vi "Hausmodell.Rücklauftemperatur.vi"(8 "Error IN":errorcluster, 10 "Vorlauftemperatur Heizkreislauf [°C]":dbl, 11 "Hausmodell IN":refnum<data-value>) -> (0 "Error OUT":errorcluster, 3 "Hausmodell OUT":refnum<data-value>)   [LabVIEW 2016, in "Hausmodell.lvclass"]
uses:
  Hausmodell.lvclass
  Hausmodell.lvclass/Hausmodell.ctl
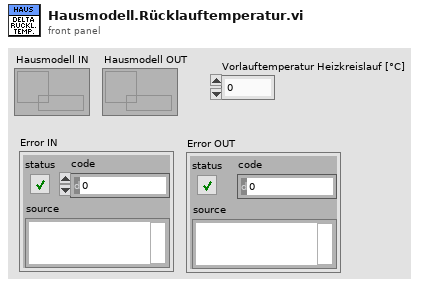
[diagram p1: front panel]
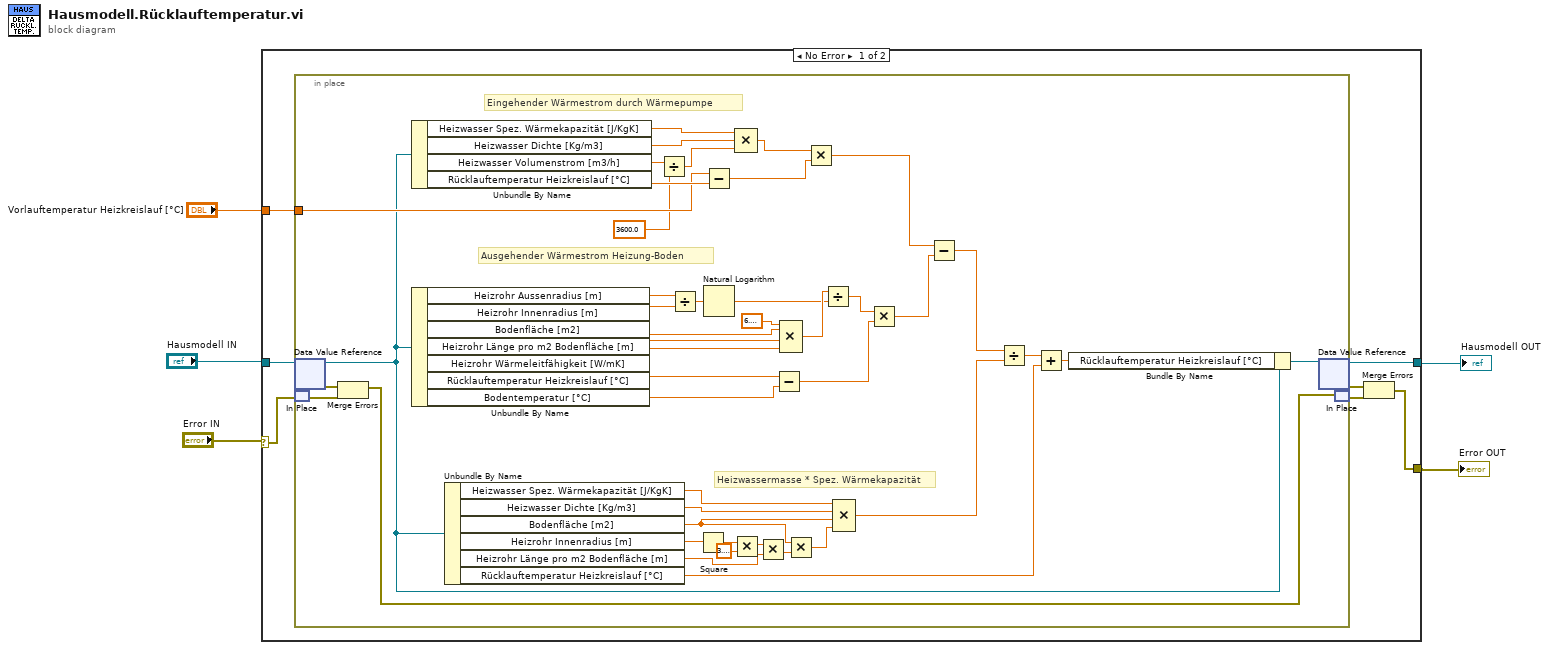
[diagram p0: block diagram]
diagram:
  n1 = case shown="No Error" "Error IN" {
    selector: "Error IN" -> [w11 w58]
    tunnel: [w12 w57] -> w3
    tunnel: [w9 w58] -> w2
    tunnel: "Hausmodell IN" -> [w7 w57]
    tunnel: "Vorlauftemperatur Heizkreislauf [°C]" -> [w6 _]
    frame No Error {
      n2 = in-place {
        in-place-border: w6 -> [w41]
        # "Heizwassermasse * Spez. Wärmekapazität"
        # "Ausgehender Wärmestrom Heizung-Boden"
        # "Eingehender Wärmestrom durch Wärmepumpe"
        n3 = in-place-dvr #1(w7) -> (w29:refnum<class "Hausmodell.lvclass">, w55:errorcluster)
        n4 = in-place-match #2(w11) -> (w54:errorcluster)
        n5 = Merge Errors(w55, w54) -> (w53:errorcluster)
        n6 = Unbundle By Name(w29) -> ("Heizwasser Spez. Wärmekapazität [J/KgK]"=w45:dbl, "Heizwasser Dichte [Kg/m3]"=w44:dbl, "Heizwasser Volumenstrom [m3/h]"=w16:dbl, "Rücklauftemperatur Heizkreislauf [°C]"=w43:dbl)
        n7 = Unbundle By Name(w29) -> ("Heizrohr Aussenradius [m]"=w34:dbl, "Heizrohr Innenradius [m]"=w33:dbl, "Bodenfläche [m2]"=w32:dbl, "Heizrohr Länge pro m2 Bodenfläche [m]"=w31:dbl, "Heizrohr Wärmeleitfähigkeit [W/mK]"=w30:dbl, "Rücklauftemperatur Heizkreislauf [°C]"=w28:dbl, "Bodentemperatur [°C]"=w27:dbl)
        n8 = Unbundle By Name(w29) -> ("Heizwasser Spez. Wärmekapazität [J/KgK]"=w48:dbl, "Heizwasser Dichte [Kg/m3]"=w47:dbl, "Bodenfläche [m2]"=w18:dbl, "Heizrohr Innenradius [m]"=w24:dbl, "Heizrohr Länge pro m2 Bodenfläche [m]"=w20:dbl, "Rücklauftemperatur Heizkreislauf [°C]"=w25:dbl)
        n9 = Divide(x=w16, y=3600.0) -> (x/y=w14:dbl)
        n10 = Divide(x=w34, y=w33) -> (x/y=w40:dbl)
        n11 = Square(x=w24) -> (x^2=w23:dbl)
        n12 = Subtract(x=w41, y=w43) -> (x-y=w42:dbl)
        n13 = Natural Logarithm(1:w40) -> (0:w36:dbl)
        n14 = Multiply(x=w23, y=3.141592653589793) -> (x*y=w21:dbl)
        n15 = Compound Arithmetic op=MULTIPLY(w45, w44, w14) -> (w13:dbl)
        n16 = Multiply(x=w21, y=w20) -> (x*y=w19:dbl)
        n17 = Subtract(x=w28, y=w27) -> (x-y=w35:dbl)
        n18 = Compound Arithmetic op=MULTIPLY(6.283185307179586, w32, w31, w30) -> (w37:dbl)
        n19 = Multiply(x=w18, y=w19) -> (x*y=w17:dbl)
        n20 = Multiply(x=w13, y=w42) -> (x*y=w52:dbl)
        n21 = Divide(x=w37, y=w36) -> (x/y=w38:dbl)
        n22 = Compound Arithmetic op=MULTIPLY(w48, w47, w18, w17) -> (w46:dbl)
        n23 = Multiply(x=w38, y=w35) -> (x*y=w26:dbl)
        n24 = Subtract(x=w52, y=w26) -> (x-y=w51:dbl)
        n25 = Divide(x=w51, y=w46) -> (x/y=w50:dbl)
        n26 = Add(x=w50, y=w25) -> (x+y=w49:dbl)
        n27 = Bundle By Name(cluster=w29, "Rücklauftemperatur Heizkreislauf [°C]"=w49) -> (w56:refnum<class "Hausmodell.lvclass">)
        n28 = in-place-dvr #1(w56) -> (w12:refnum<data-value>, w10:errorcluster)
        n29 = in-place-match #2(w53) -> (w8:errorcluster)
      }
      n30 = Merge Errors(w10, w8) -> (w9:errorcluster)
    }
    frame Error {
    }
  }
  "Hausmodell OUT" <- w3
  "Error OUT" <- w2
